vi "String to Response Header.vi"(8 "error in (no error)":errorcluster, 9 "body":string, 10 "headers":string, 11 "http-client in":refnum<class "basic-http-client.lvclass">) -> (0 "error out":errorcluster, 2 "response":refnum<class "response.lvclass">, 3 "http-client out":refnum<class "basic-http-client.lvclass">)   [LabVIEW 2020, in "http.lvlib"]
uses:
  http.lvlib
  response/response.lvclass
  basic-http-client/basic-http-client.lvclass
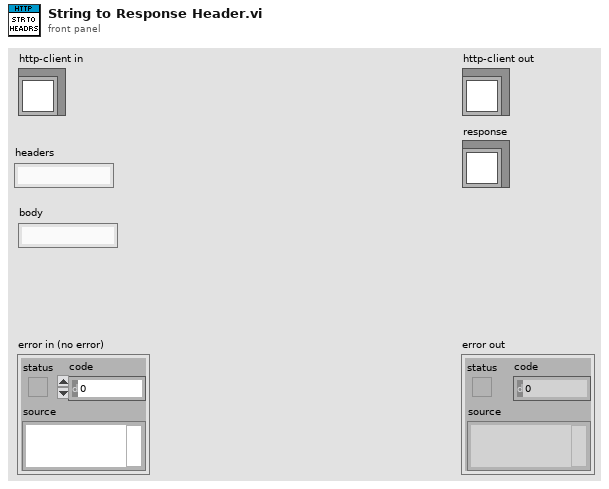
[diagram p1: front panel]
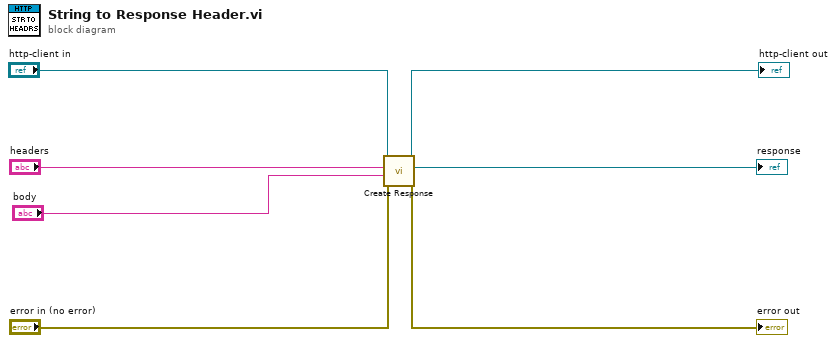
[diagram p0: block diagram]
diagram:
  n1 = call-dynamic "Create Response.vi"("error in (no error)"="error in (no error)", "body"="body", "headers"="headers", "http-client"="http-client in") -> ("error out"=→"error out":errorcluster, "response"=→"response":refnum<class "response.lvclass">, "http-client out"=→"http-client out":refnum<class "basic-http-client.lvclass">)  [unwired: 5 in]
